vi "TopHat.vi"(11 "General settings":T1) -> (2 "TopHat":dbl[][](array[numeric]))   [LabVIEW 2018]
uses:
  Controls/General Setting.ctl
  Controls/Buttons/Running Button.ctl
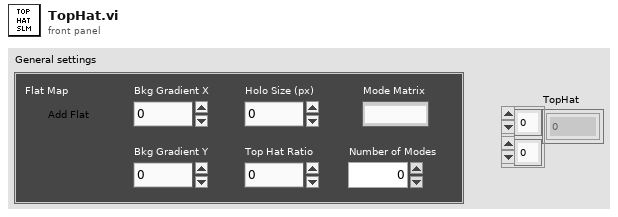
[diagram p1: front panel]
types:
  T1 = typedef "General Setting.ctl" = cluster{"Flat Map":T2, "Bkg Gradient X":dbl, "Bkg Gradient Y":dbl, "Holo Size (px)":i32, "Top Hat Ratio":dbl, "Number of Modes":i8, "Mode Matrix":u16}
  T2 = typedef "Running Button.ctl" = bool
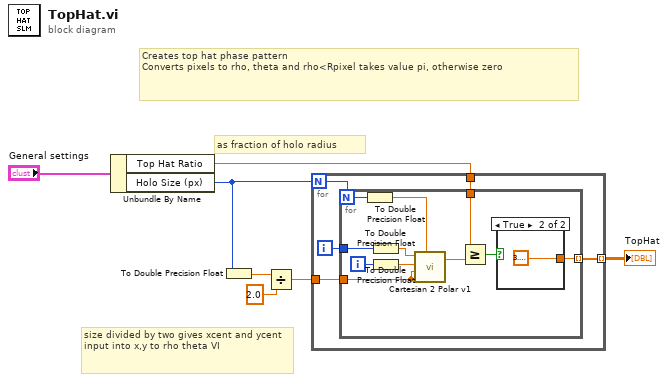
[diagram p0: block diagram]
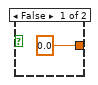
[diagram p2: hidden frame]
diagram:
  # "as fraction of holo radius"
  # "Creates top hat phase pattern\nConverts pixels to rho, theta and rho<Rpixel takes value pi, otherwise zero"
  # "size divided by two gives xcent and ycent input into x,y to rho theta VI"
  n1 = Unbundle By Name("General settings") -> ("Top Hat Ratio"=w1:dbl, "Holo Size (px)"=w3:i32)
  n2 = To Double Precision Float(number=w3) -> (double precision float=w2:dbl)
  n3 = Divide(x=w2, y=2.0) -> (x/y=w5:dbl)
  n4 = for {
    N: w3 -> [w9]
    tunnel: [w11] -> w6 mode=indexing
    tunnel: w5 -> [w10]
    tunnel: w1 -> [w8]
    i -> [w12]
    n5 = for {
      N: w9 -> [w18]
      tunnel: w12 -> [w22]
      tunnel: [w17] -> w11 mode=indexing
      tunnel: w10 -> [w19]
      tunnel: w8 -> [w16]
      i -> [w23]
      n6 = To Double Precision Float(number=w18) -> (double precision float=w15:dbl)
      n7 = To Double Precision Float(number=w22) -> (double precision float=w14:dbl)
      n8 = To Double Precision Float(number=w23) -> (double precision float=w13:dbl)
      n9 = call "Cartesian 2 Polar v1.vi"("x"=w14, "y"=w13, "xcent"=w19, "ycent"=w19, "diam"=w15) -> ("rho"=w20:dbl)  [unwired: 1 out]
      n10 = Greater Or Equal?(x=w16, y=w20) -> (x >= y?=w21:bool)
      n11 = case shown="True" w21 {
        tunnel: [0.0 ("zernike") 3.141592653589793] -> w17
        frame False {
        }
        frame True {
        }
      }
    }
  }
  "TopHat" <- w6
